vi "Get Run Ref.vi"(8 "error in (no error)":errorcluster, 11 "xwpfRun in":refnum<class "xwpfRun.lvclass">) -> (0 "error out":errorcluster, 2 "Run Ref":refnum<k24>, 3 "xwpfRun out":refnum<class "xwpfRun.lvclass">)   [LabVIEW 2017, in "Word_Specific.lvlib" / "xwpfRun.lvclass"]
uses:
  xwpfRun.lvclass
  C:/Users/Neo/Desktop/Dev_Tools_BR/LabVIEW_NPOI/src/lib/NPOI 2.1.1/NPOI.OOXML.dll
  lib/NPOI 2.1.1/NPOI.OOXML.dll
  xwpfRun.lvclass/xwpfRun.ctl
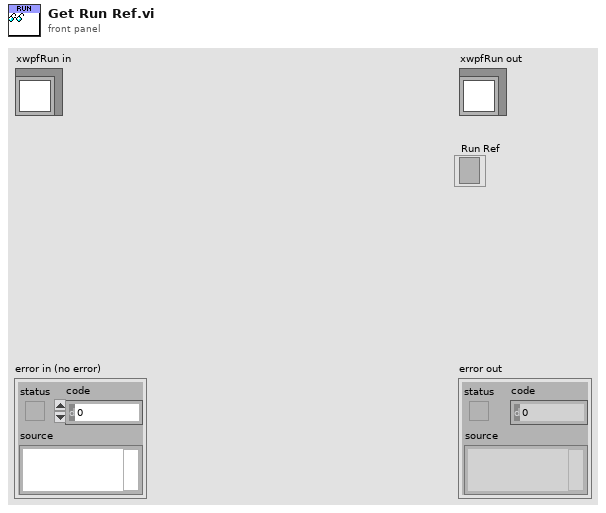
[diagram p1: front panel]
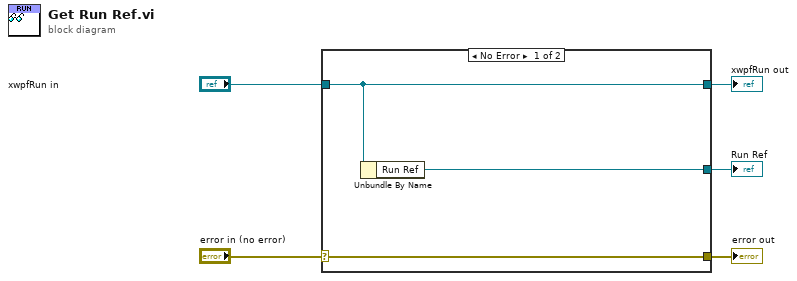
[diagram p0: block diagram]
diagram:
  n1 = case shown="No Error" "error in (no error)" {
    selector: "error in (no error)" -> [w8 w9]
    tunnel: [w8 w9] -> w4
    tunnel: [w7 w10] -> w2
    tunnel: "xwpfRun in" -> [w7 w10]
    tunnel: [w6 _] -> w1
    frame No Error {
      n2 = Unbundle By Name(w7) -> ("Run Ref"=w6:refnum<k24>)
    }
    frame Error {
    }
  }
  "error out" <- w4
  "xwpfRun out" <- w2
  "Run Ref" <- w1
